vi "MCLB_ItemName_Tests.vi"(11 "error in":errorcluster) -> (15 "error out":errorcluster)   [LabVIEW 2016, in "DronaTest.lvlib"]
uses:
  DronaTest.lvlib
  APIs/Stimulus/ControlValue/SetValueAuto.vi
  APIs/Stimulus/ControlValue/Controls/MC Listbox/SetValueByItemName.vi
  APIs/Assert/AssertControlValue/Equal.vi
  <vilib>/addons/_JKI Toolkits/Caraya/classes/Assert/Assert Equal Value_Variant.vi
  APIs/Get/GetControlRef/GetControlRefByPath.vi
  <vilib>/addons/_JKI Toolkits/Caraya/classes/Test/Test.lvclass
  Drona.lvlib
  <vilib>/SLL Toolkit/SLL Debug/SLL Debug.lvlib
  APIs/Assert/AssertControlValue/AssertControlValue.lvlib
  APIs/Stimulus/ControlValue/ControlValue.lvlib
  <vilib>/addons/_JKI Toolkits/Caraya/classes/Assert/Assert.lvclass
  APIs/Stimulus/ControlValue/Controls/MC Listbox/StimulusMCListbox.lvlib
  APIs/Get/GetControlRef/GetControlRef.lvlib
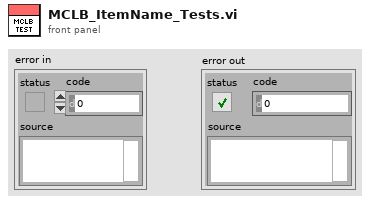
[diagram p1: front panel]
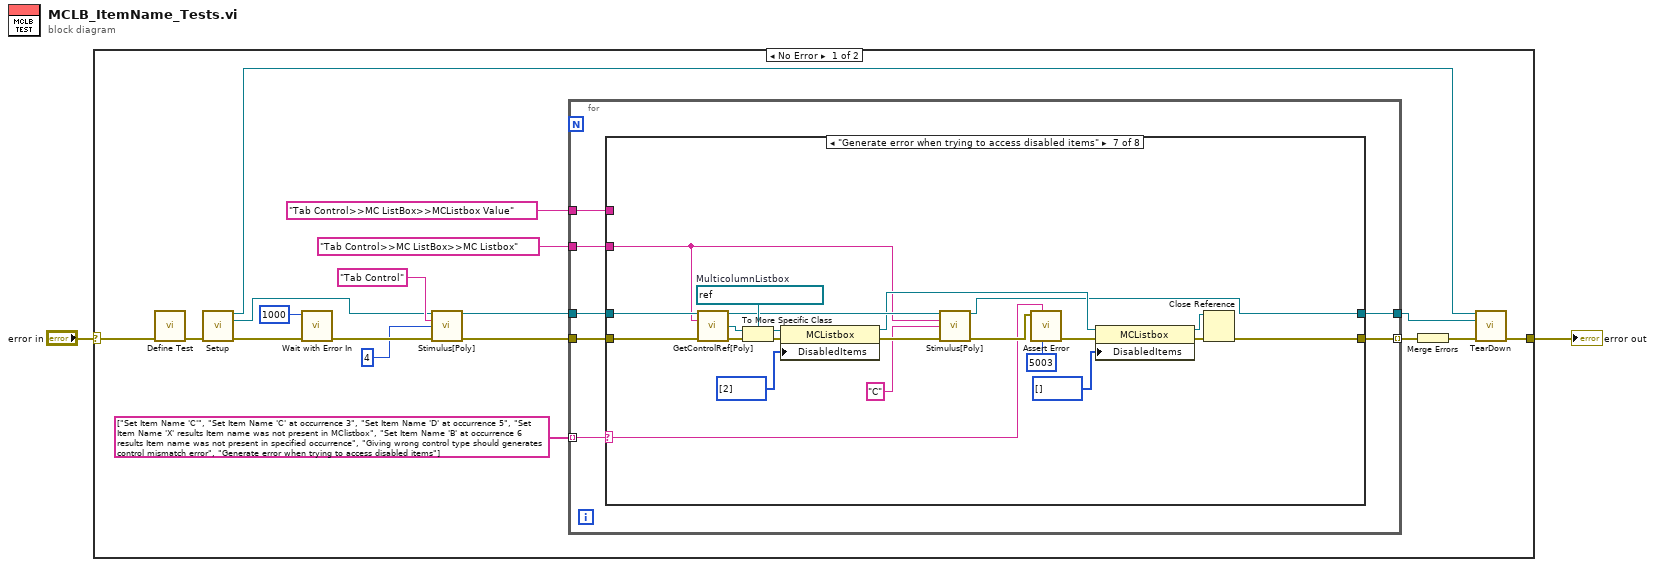
[diagram p0: block diagram]
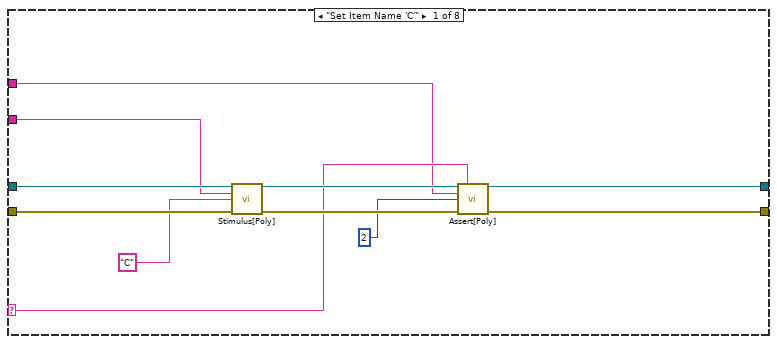
[diagram p2: hidden frame]
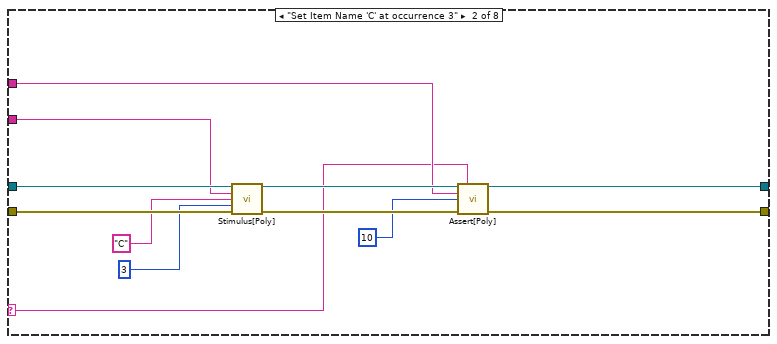
[diagram p3: hidden frame]
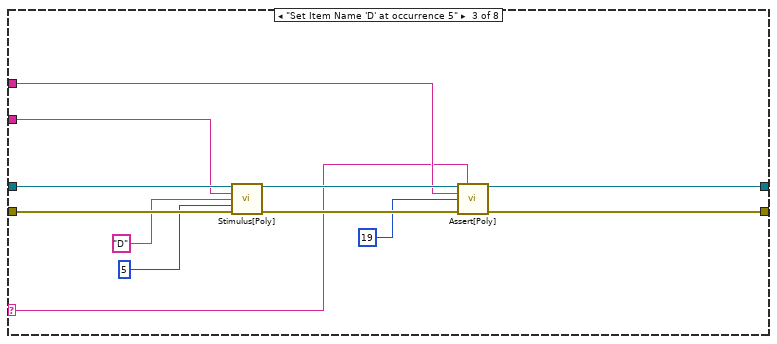
[diagram p4: hidden frame]
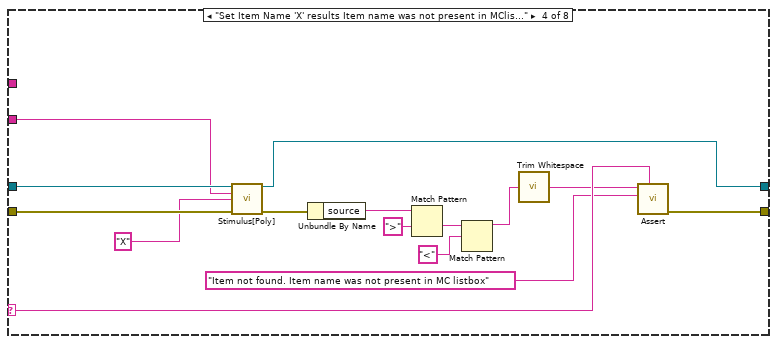
[diagram p5: hidden frame]
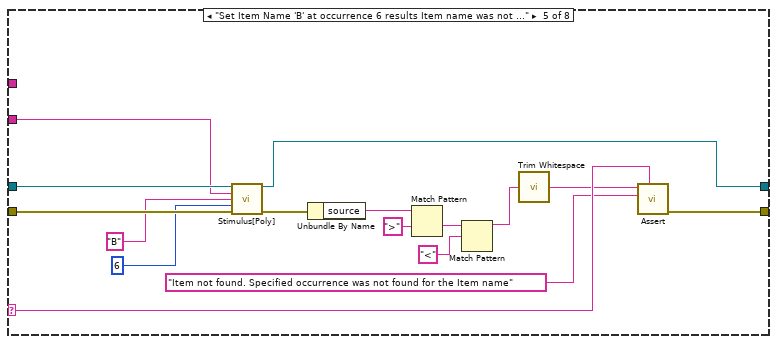
[diagram p6: hidden frame]
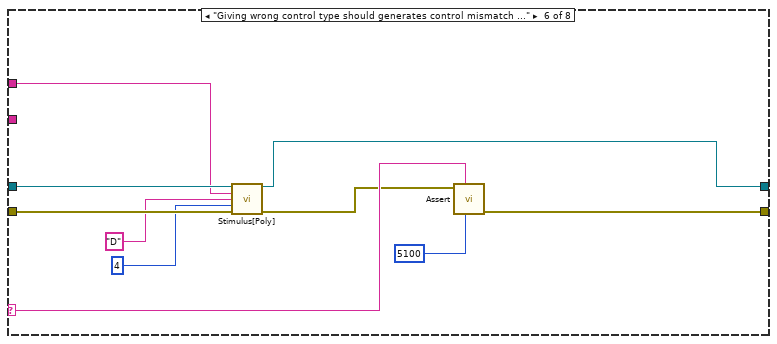
[diagram p7: hidden frame]
diagram:
  n1 = case shown="No Error" "error in" {
    selector: "error in" -> [w20 w128]
    tunnel: [w3 w128] -> w1
    frame No Error {
      n2 = call <vilib>:"Define Test.vi"("error in (no error)"=w20) -> ("error out"=w9:errorcluster)  [unwired: 9 in, 1 out]
      n3 = call "Setup.vi"("error in"=w9) -> ("Application Ref"=w4:refnum<vi>, "VI out"=w8:refnum<vi>, "error out"=w7:errorcluster)  [unwired: 12 in]
      n4 = call <vilib>:"Wait with Error In.vi"("error in (no error)"=w7, "milliseconds to wait"=u32 1000) -> ("error out"=w18:errorcluster)  [unwired: 9 in]
      n5 = call-poly "Stimulus[Poly].vi"("VI Reference In"=w8, "Control Path"="Tab Control", "Value (Signaling)"=4, "error in"=w18) -> ("VI Reference Out"=w14:refnum<vi>, "error out"=w17:errorcluster)  [unwired: 10 in]
      n6 = for {
        tunnel: w14 -> [w26]
        tunnel: "Tab Control>>MC ListBox>>MC Listbox" ("Control Path") -> [w25]
        tunnel: "Tab Control>>MC ListBox>>MCListbox Value" ("Control Path") -> [w24]
        tunnel: string[] ["Set Item Name 'C'", "Set Item Name 'C' at occurrence 3", "Set Item Name 'D' at occurrence 5", "Set Item Name 'X' results Item name was not present in MClistbox", "Set Item Name 'B' at occurrence 6 results Item name was not present in specified occurrence", "Giving wrong control type should generates control mismatch error", "Generate error when trying to access disabled items"] -> [w22] mode=indexing
        tunnel: [w21] -> w5
        tunnel: w17 -> [w27]
        tunnel: [w23] -> w10 mode=indexing
        n7 = case shown="\"Generate error when trying to access disabled items\"" w22 {
          selector: w22 -> [w32 w42 w54 w73 w89 w100 w106 _]
          tunnel: w27 -> [w38 w50 w62 w77 w93 w103 w109 w127]
          tunnel: w26 -> [w37 w49 w61 w76 w92 w102 w105 w126]
          tunnel: w25 -> [w28 w46 w58 w75 w91 _ w104 _]
          tunnel: w24 -> [w29 w45 w57 _ _ w94 _ _]
          tunnel: [w34 w44 w56 w74 w90 w101 w108 w127] -> w23
          tunnel: [w33 w43 w55 w72 w88 w99 w107 w126] -> w21
          frame "Set Item Name 'C'" {
            n8 = call-poly "Stimulus[Poly].vi"("VI Reference In"=w37, "Control Path"=w28, "Item Name"="C", "Error In"=w38) -> ("VI Reference Out"=w35:refnum<vi>, "Error Out"=w36:errorcluster)  [unwired: 10 in]
            n9 = call-poly "Assert[Poly].vi"("VI Reference In"=w35, "Test Label"=w32, "Control Path"=w29, "Control Value"=2, "Error In"=w36) -> ("VI Reference Out"=w33:refnum<vi>, "Error Out"=w34:errorcluster)  [unwired: 8 in, 1 out]
          }
          frame "Set Item Name 'C' at occurrence 3" {
            n10 = call-poly "Stimulus[Poly].vi"("VI Reference In"=w49, "Control Path"=w46, "Item Name"="C", "Occurrence"=3, "Error In"=w50) -> ("VI Reference Out"=w47:refnum<vi>, "Error Out"=w48:errorcluster)  [unwired: 9 in]
            n11 = call-poly "Assert[Poly].vi"("VI Reference In"=w47, "Test Label"=w42, "Control Path"=w45, "Control Value"=10, "Error In"=w48) -> ("VI Reference Out"=w43:refnum<vi>, "Error Out"=w44:errorcluster)  [unwired: 8 in, 1 out]
          }
          frame "Set Item Name 'D' at occurrence 5" {
            n12 = call-poly "Stimulus[Poly].vi"("VI Reference In"=w61, "Control Path"=w58, "Item Name"="D", "Occurrence"=5, "Error In"=w62) -> ("VI Reference Out"=w59:refnum<vi>, "Error Out"=w60:errorcluster)  [unwired: 9 in]
            n13 = call-poly "Assert[Poly].vi"("VI Reference In"=w59, "Test Label"=w54, "Control Path"=w57, "Control Value"=19, "Error In"=w60) -> ("VI Reference Out"=w55:refnum<vi>, "Error Out"=w56:errorcluster)  [unwired: 8 in, 1 out]
          }
          frame "Set Item Name 'X' results Item name was not present in MClistbox" {
            n14 = call-poly "Stimulus[Poly].vi"("VI Reference In"=w76, "Control Path"=w75, "Item Name"="X", "Error In"=w77) -> ("VI Reference Out"=w72:refnum<vi>, "Error Out"=w70:errorcluster)  [unwired: 10 in]
            n15 = Unbundle By Name(w70) -> ("source"=w68:string)
            n16 = Match Pattern(string=w68, regular expression=">") -> (after substring=w66:string)  [unwired: 1 in, 3 out]
            n17 = Match Pattern(string=w66, regular expression="<") -> (before substring=w64:string)  [unwired: 1 in, 3 out]
            n18 = call <vilib>:"Trim Whitespace.vi"("string"=w64) -> ("trimmed string"=w63:string)  [unwired: 1 in]
            n19 = call-poly <vilib>:"Assert.vi"("Label"=w73, "Y"="Item not found. Item name was not present in MC listbox", "X"=w63) -> ("error out"=w74:errorcluster)  [unwired: 7 in, 1 out]
          }
          frame "Set Item Name 'B' at occurrence 6 results Item name was not present in specified occurrence" {
            n20 = call-poly "Stimulus[Poly].vi"("VI Reference In"=w92, "Control Path"=w91, "Item Name"="B", "Occurrence"=6, "Error In"=w93) -> ("VI Reference Out"=w88:refnum<vi>, "Error Out"=w86:errorcluster)  [unwired: 9 in]
            n21 = Unbundle By Name(w86) -> ("source"=w84:string)
            n22 = Match Pattern(string=w84, regular expression=">") -> (after substring=w82:string)  [unwired: 1 in, 3 out]
            n23 = Match Pattern(string=w82, regular expression="<") -> (before substring=w80:string)  [unwired: 1 in, 3 out]
            n24 = call <vilib>:"Trim Whitespace.vi"("string"=w80) -> ("trimmed string"=w79:string)  [unwired: 1 in]
            n25 = call-poly <vilib>:"Assert.vi"("Label"=w89, "Y"="Item not found. Specified occurrence was not found for the Item name", "X"=w79) -> ("error out"=w90:errorcluster)  [unwired: 7 in, 1 out]
          }
          frame "Giving wrong control type should generates control mismatch error" {
            n26 = call-poly "Stimulus[Poly].vi"("VI Reference In"=w102, "Control Path"=w94, "Item Name"="D", "Occurrence"=4, "Error In"=w103) -> ("VI Reference Out"=w99:refnum<vi>, "Error Out"=w96:errorcluster)  [unwired: 9 in]
            n27 = call-poly <vilib>:"Assert.vi"("error code (1)"=5100, "Label"=w100, "Error?"=w96) -> ("error out"=w101:errorcluster)  [unwired: 7 in, 1 out]
          }
          frame "Generate error when trying to access disabled items" {
            w122 = refnum<vi> refnum  # MulticolumnListbox
            n28 = call-poly "GetControlRef[Poly].vi"("VI Reference In"=w105, "Control Path"=w104, "error In"=w109) -> ("VI Reference Out"=w118:refnum<vi>, "Ctl Refnum"=w123:refnum<vi>, "error out"=w125:errorcluster)  [unwired: 10 in]
            n29 = To More Specific Class(target class=w122, reference=w123, error in=w125) -> (specific class reference=w121:refnum<vi>, error out=w124:errorcluster)
            n30 = property class="MCListbox"(reference=w121, error in=w124, "DisabledItems"=i32[] [2] ("Disabled Items")) -> (reference out=w115:refnum<vi>, error out=w119:errorcluster)
            n31 = call-poly "Stimulus[Poly].vi"("VI Reference In"=w118, "Control Path"=w104, "Item Name"="C" ("Item Index"), "Error In"=w119) -> ("VI Reference Out"=w107:refnum<vi>, "Error Out"=w112:errorcluster)  [unwired: 10 in]
            n32 = call <vilib>:"Assert Error.vi"("error code (1)"=5003, "Label"=w106, "Error?"=w112) -> ("error out"=w111:errorcluster)  [unwired: 7 in, 1 out]
            n33 = property class="MCListbox"(reference=w115, error in=w111, "DisabledItems"=i32[] [] ("Disabled Items")) -> (reference out=w113:refnum<vi>, error out=w116:errorcluster)
            n34 = Close Reference(reference=w113, error in (no error)=w116) -> (error out=w108:errorcluster)
          }
          frame Default {
          }
        }
      }
      n35 = Merge Errors(w10) -> (w6:errorcluster)
      n36 = call "TearDown.vi"("Application Ref"=w4, "VI in"=w5, "error in (no error)"=w6) -> ("error out"=w3:errorcluster)  [unwired: 12 in]
    }
    frame Error {
    }
  }
  "error out" <- w1
